vi "getSingleToneData.vi"(8 "error in (no error)":errorcluster, 11 "rf in":refnum<class "rf.lvclass">) -> (0 "error out":errorcluster, 1 "amplitude":dbl, 2 "time":dbl, 3 "rf out":refnum<class "rf.lvclass">, 4 "frequency":dbl, 5 "phase":dbl)   [LabVIEW 2009, in "Tools.lvlib" / "Scripting.lvlib" / "rf.lvclass"]
uses:
  rf.lvclass
  rf.lvclass/rf.ctl
  ScriptEvent.lvclass
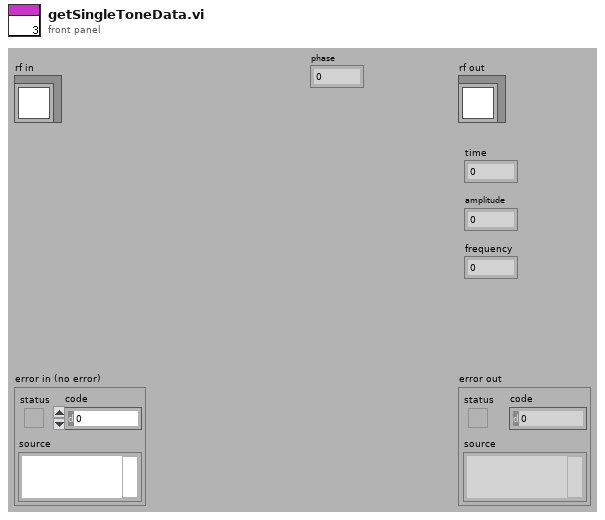
[diagram p1: front panel]
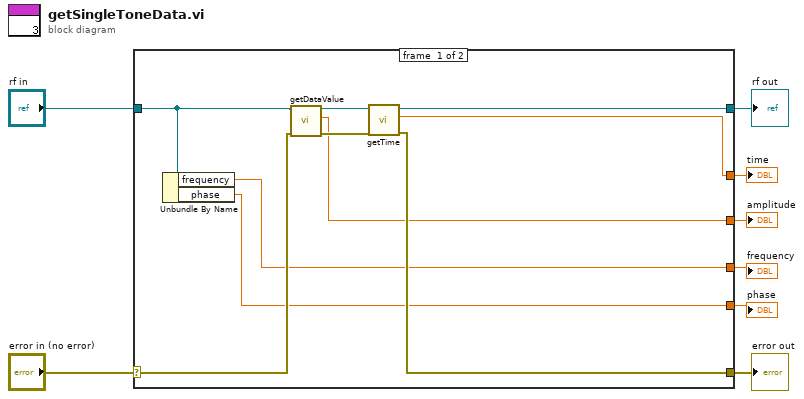
[diagram p0: block diagram]
diagram:
  n1 = case shown="No Error" "error in (no error)" {
    selector: "error in (no error)" -> [w17 w20]
    tunnel: [w13 w20] -> w7
    tunnel: [w14 w19] -> w5
    tunnel: "rf in" -> [w18 w19]
    tunnel: [w12 _] -> w4
    tunnel: [w11 _] -> w3
    tunnel: [w10 _] -> w2
    tunnel: [w9 _] -> w1
    frame #0 {
      n2 = Unbundle By Name(w18) -> ("frequency"=w10:dbl, "phase"=w9:dbl)
      n3 = call "getDataValue.vi"("error in (no error)"=w17, "ScriptEvent.lvclass in"=w18) -> ("error out"=w15:errorcluster, "dataValue"=w11:dbl, "ScriptEvent.lvclass out"=w16:refnum<class "rf.lvclass">)  [unwired: 7 in]
      n4 = call "getTime.vi"("error in (no error)"=w15, "ScriptEvent.lvclass in"=w16) -> ("error out"=w13:errorcluster, "time"=w12:dbl, "ScriptEvent.lvclass out"=w14:refnum<class "rf.lvclass">)  [unwired: 7 in]
    }
    frame #1 {
    }
  }
  "error out" <- w7
  "rf out" <- w5
  "time" <- w4
  "amplitude" <- w3
  "frequency" <- w2
  "phase" <- w1
